vi "Config Spectrometer.vi"(6 "Ref Lvl Auto":bool, 7 "Valor de Span (nm)":dbl=100.0, 8 "error in (no error)":errorcluster, 9 "Centro do Pico do espectro (nm)":dbl=1550.0, 10 "Resolution":enum16{"Normal", "High"}(ring), 11 "VISA Refnum in":refnum<visa-resource-name>="GPIB0::9::INSTR") -> (0 "error out":errorcluster, 3 "VISA Refnum out":refnum<visa-resource-name>)   [LabVIEW 2018]
uses:
  f45516d5-78c5-4aba-88ba-dcf34f3dc23c.vi
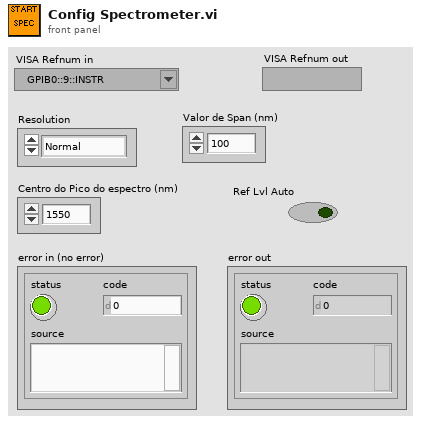
[diagram p1: front panel]
types:
  T1 = enum16{"um", "nm", "nm/DIV", "mm", "THz", "GHz", "THz/DIV", "GHz/DIV"}
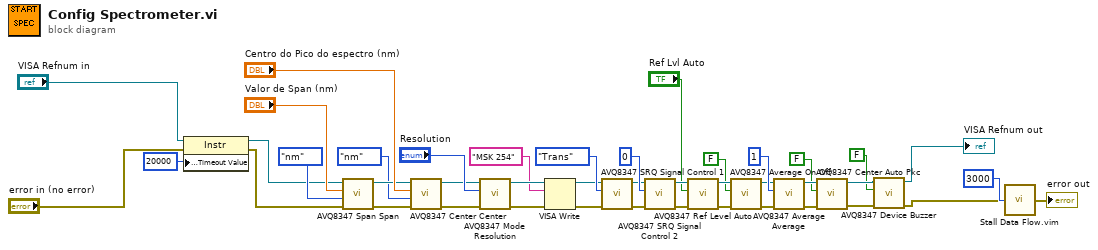
[diagram p0: block diagram]
diagram:
  n1 = property class="Instr"(reference="VISA Refnum in", error in="error in (no error)", "General Settings:Timeout Value"=u32 20000) -> (reference out=w8:refnum<visa-resource-name>, error out=w7:errorcluster)
  n2 = call "AVQ8347 Span Span.vi"("Error In"=w7, "Span Unit (nm)"=T1."nm", "Span Value (700)"="Valor de Span (nm)", "VISA Session"=w8) -> ("Error Out"=w33:errorcluster, "Copy VISA Session"=w34:refnum<visa-resource-name>)  [unwired: 5 in, 1 out]
  n3 = call "AVQ8347 Center Center.vi"("Error In"=w33, "Center Point Unit (nm)"=enum16{"um", "nm", "THz", "GHz"}."nm", "Center Point Value (700)"="Centro do Pico do espectro (nm)", "VISA Session"=w34) -> ("Error Out"=w31:errorcluster, "Copy VISA Session"=w30:refnum<visa-resource-name>)  [unwired: 5 in, 1 out]
  n4 = call "AVQ8347 Mode Resolution.vi"("Error In"=w31, "Mode Select (Normal)"="Resolution", "VISA Session"=w30) -> ("Error Out"=w28:errorcluster, "Copy VISA Session"=w29:refnum<visa-resource-name>)  [unwired: 6 in, 1 out]
  n5 = VISA Write(VISA resource name=w29, write buffer="MSK 254", error in (no error)=w28) -> (VISA resource name out=w15:refnum<visa-resource-name>, error out=w14:errorcluster)  [unwired: 1 out]
  n6 = call "AVQ8347 SRQ Signal Control 1.vi"("Error In"=w14, "SRQ Trans Sel (No Trans)"=enum16{"No Trans", "Trans"}."Trans", "VISA Session"=w15) -> ("Error Out"=w12:errorcluster, "Copy VISA Session"=w13:refnum<visa-resource-name>)  [unwired: 6 in, 1 out]
  n7 = call "AVQ8347 SRQ Signal Control 2.vi"("Error In"=w12, "SRQ Trans Sel (No Trans)"=u16 0 ("Average Value (1)"), "VISA Session"=w13) -> ("Error Out"=w40:errorcluster, "Copy VISA Session"=w39:refnum<visa-resource-name>)  [unwired: 6 in, 1 out]
  n8 = call "AVQ8347 Ref Level Auto.vi"("Error In"=w40, "Mode selection (OFF)"="Ref Lvl Auto", "VISA Session"=w39) -> ("Error Out"=w24:errorcluster, "Copy VISA Session"=w25:refnum<visa-resource-name>)  [unwired: 6 in, 1 out]
  n9 = call "AVQ8347 Average On Off.vi"("Error In"=w24, "Processing Select (OFF)"=FALSE, "VISA Session"=w25) -> ("Error Out"=w23:errorcluster, "Copy VISA Session"=w22:refnum<visa-resource-name>)  [unwired: 6 in, 1 out]
  n10 = call "AVQ8347 Average Average.vi"("Error In"=w23, "Average Value (1)"=u16 1, "VISA Session"=w22) -> ("Error Out"=w19:errorcluster, "Copy VISA Session"=w20:refnum<visa-resource-name>)  [unwired: 6 in, 1 out]
  n11 = call "AVQ8347 Center Auto Pkc.vi"("Error In"=w19, "APC Function selection (OFF)"=FALSE, "VISA Session"=w20) -> ("Error Out"=w6:errorcluster, "Copy VISA Session"=w3:refnum<visa-resource-name>)  [unwired: 6 in, 1 out]
  n12 = call "AVQ8347 Device Buzzer.vi"("Error In"=w6, "Buzzer Control (OFF)"=FALSE, "VISA Session"=w3) -> ("Error Out"=w5:errorcluster, "Copy VISA Session"=→"VISA Refnum out":refnum<visa-resource-name>)  [unwired: 6 in, 1 out]
  n13 = call "Stall Data Flow.vim"("value in"=w5, "milliseconds to wait"=u32 3000) -> ("value out"=→"error out":errorcluster)  [unwired: 1 out]
